vi "Read Base Actor.vi"(11 "TEMPLATE Actor in":refnum<class "TEMPLATE Actor.lvclass">) -> (2 "Base Actor":refnum<data-value>)   [LabVIEW 2020, in "_Template.lvlib" / "Templates.lvlib" / "TEMPLATE jettl Actor.lvlib" / "TEMPLATE Actor.lvlib" / "TEMPLATE Actor.lvclass"]
uses:
  TEMPLATE Actor.lvclass
  TEMPLATE Actor.lvclass/TEMPLATE Actor.ctl
  jettl/jettl/jettl.lvlib
  jettl/jettl/Lifetime.ctl
  jettl/jettl/Base Actor.ctl
panel:
  # "This front panel should not be manipulated."
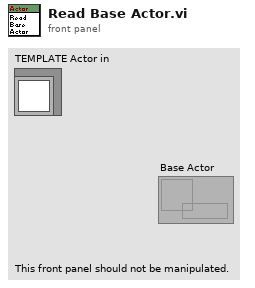
[diagram p1: front panel]
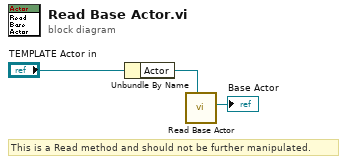
[diagram p0: block diagram]
diagram:
  # "This is a Read method and should not be further manipulated."
  n1 = Unbundle By Name("TEMPLATE Actor in") -> ("Actor"=w1:refnum<data-value>)
  n2 = call "Read Base Actor.vi"("Actor in"=w1) -> ("Base Actor"=→"Base Actor":refnum<data-value>)  [unwired: 9 in, 1 out]
